vi "Application Example Advanced with Debug.vi"() -> ()   [LabVIEW 2019]
uses:
  <vilib>/addons/Automotive Diagnostic Command Set/NI_Automotive Diagnostic Command Set.lvlib
  Engine/SubVIs/GMLAN/GMLAN.lvlib
  Engine/SubVIs/GMLAN/_SubVIs/ReadDiagnosticInformation_ByStatus.vi
  <vilib>/xnet/xnet.llb/XNET Frame Type CAN.ctl
  <vilib>/xnet/xnet.llb/XNET Frame CAN.ctl
  <vilib>/Automotive Diagnostic Command Set/Diagnostic Transport.llb/Property ID.ctl
  Engine/SubVIs/GMLAN/_SubVIs/ReadDataByPacketIdentifier_SubFunctions.ctl
  <vilib>/Automotive Diagnostic Command Set/Diagnostic Transport.llb/Transport Protocol Selector.ctl
  Engine/SubVIs/GMLAN/_SubVIs/DisableNormalCommunication_Parameter.ctl
  <vilib>/xnet/xnet.llb/XNET Database Close (Database).vi
  <vilib>/xnet/xnet.llb/XNET Read (Frame CAN).vi
  <vilib>/xnet/xnet.llb/XNET Create Session (Frame Input Queued).vi
  <vilib>/Automotive Diagnostic Command Set/Diagnostic Protocols.llb/Diagnostic Trouble Code.ctl
  <vilib>/Automotive Diagnostic Command Set/Diagnostic Transport.llb/Diag CAN Frame Log.ctl
  <resource>/objmgr/xnet.rc
  _SubVIs/CAN Frame.ctl
  <vilib>/Automotive Diagnostic Command Set/Diagnostic Protocols.llb/DTC Descriptor.ctl
  _SubVIs/DPID Periodic Rate.ctl
  _SubVIs/DPID Parameters.ctl
  Engine/SubVIs/GMLAN/_SubVIs/DTCStatusMask.ctl
panel:
  in  "Enable Comm":bool
  out "Bus Traffic":string[][](table)=[["09/16/2012 22:50:39.244581", "01\t68\tAA\tAA\tAA\tAA\tAA\tAA\r\n", "000007E8", "CAN Data", "No", "No"], ["09/16/2012 22:50:39.235716", "ED\t40\t00\t0F\t38\t00\t83\tFD\r\n", "000001F5", "CAN Data", "No", "No"], ["09/16/2012 22:50:39.235476", "6D\t02\tC0\t30\r\n", "000001C4", "CAN Data", "No", "No"], ["09/16/2012 22:50:39.235306", "06\t45\t07\t06\t00\t00\t00\t00\r\n", "000001C3", "CAN Data", "No", "No"], ["09/16/2012 22:50:39.234921", "00\t00\t00\t00\r\n", "000001EF", "CAN Data", "No", "No"], ["09/16/2012 22:50:39.234745", "01\t90\t00\t00\t00\t00\t00\t00\r\n", "000001ED", "CAN Data", "No", "No"], ["09/16/2012 22:50:39.234497", "00\t00\t00\t0D\t00\t10\t00\t00\r\n", "000000C9", "CAN Data", "No", "No"], ["09/16/2012 22:50:39.222361", "00\t00\t00\t00\r\n", "000001EF", "CAN Data", "No", "No"], ["09/16/2012 22:50:39.222179", "01\t90\t00\t00\t00\t00\t00\t00\r\n", "000001ED", "CAN Data", "No", "No"], ["09/16/2012 22:50:39.221930", "00\t00\t00\t0A\t00\t10\t00\t00\r\n", "000000C9", "CAN Data", "No", "No"], ["09/16/2012 22:50:39.211623", "00\t00\t00\t00\t00\t00\t00\t00\r\n", "000003E9", "CAN Data", "No", "No"], ["09/16/2012 22:50:39.211370", "01\t34\t00\t00\t00\t00\t00\t00\r\n", "000003D1", "CAN Data", "No", "No"], ["09/16/2012 22:50:39.211122", "07\t65\t08\t04\t00\t00\t00\t00\r\n", "000003C1", "CAN Data", "No", "No"], ["09/16/2012 22:50:39.210879", "06\t45\t06\tA0\t06\tA0\tA9\r\n", "000002C3", "CAN Data", "No", "No"], ["09/16/2012 22:50:39.210661", "ED\t40\t00\t0F\t38\t00\t83\tFD\r\n", "000001F5", "CAN Data", "No", "No"], ["09/16/2012 22:50:39.210421", "4A\t02\tC0\t30\r\n", "000001C4", "CAN Data", "No", "No"], ["09/16/2012 22:50:39.210252", "06\t45\t07\t06\t00\t00\t00\t00\r\n", "000001C3", "CAN Data", "No", "No"], ["09/16/2012 22:50:39.209862", "00\t00\t00\t00\r\n", "000001EF", "CAN Data", "No", "No"], ["09/16/2012 22:50:39.209686", "01\t90\t00\t00\t00\t00\t00\t00\r\n", "000001ED", "CAN Data", "No", "No"], ["09/16/2012 22:50:39.209438", "00\t00\t00\t07\t00\t10\t00\t00\r\n", "000000C9", "CAN Data", "No", "No"], ["09/16/2012 22:50:39.197360", "00\t00\t00\t00\r\n", "000001EF", "CAN Data", "No", "No"], ["09/16/2012 22:50:39.197180", "01\t90\t00\t00\t00\t00\t00\t00\r\n", "000001ED", "CAN Data", "No", "No"], ["09/16/2012 22:50:39.196931", "00\t00\t00\t00\t00\t10\t00\t00\r\n", "000000C9", "CAN Data", "No", "No"], ["09/16/2012 22:50:39.185679", "ED\t40\t00\t0F\t38\t00\t83\tFD\r\n", "000001F5", "CAN Data", "No", "No"], ["09/16/2012 22:50:39.185439", "27\t02\tC0\t30\r\n", "000001C4", "CAN Data", "No", "No"], ["09/16/2012 22:50:39.185273", "06\t45\t07\t06\t00\t00\t00\t00\r\n", "000001C3", "CAN Data", "No", "No"], ["09/16/2012 22:50:39.184882", "00\t00\t00\t00\r\n", "000001EF", "CAN Data", "No", "No"], ["09/16/2012 22:50:39.184708", "01\t90\t00\t00\t00\t00\t00\t00\r\n", "000001ED", "CAN Data", "No", "No"], ["09/16/2012 22:50:39.184460", "00\t00\t00\t0D\t00\t10\t00\t00\r\n", "000000C9", "CAN Data", "No", "No"], ["09/16/2012 22:50:39.172360", "00\t00\t00\t00\r\n", "000001EF", "CAN Data", "No", "No"], ["09/16/2012 22:50:39.172178", "01\t90\t00\t00\t00\t00\t00\t00\r\n", "000001ED", "CAN Data", "No", "No"], ["09/16/2012 22:50:39.171929", "00\t00\t00\t0A\t00\t10\t00\t00\r\n", "000000C9", "CAN Data", "No", "No"], ["09/16/2012 22:50:39.160898", "06\t45\t06\tA0\t06\tA0\tA9\r\n", "000002C3", "CAN Data", "No", "No"], ["09/16/2012 22:50:39.160679", "ED\t40\t00\t0F\t38\t00\t83\tFD\r\n", "000001F5", "CAN Data", "No", "No"], ["09/16/2012 22:50:39.160439", "00\t02\tC0\t30\r\n", "000001C4", "CAN Data", "No", "No"], ["09/16/2012 22:50:39.160263", "06\t45\t07\t06\t00\t00\t00\t00\r\n", "000001C3", "CAN Data", "No", "No"], ["09/16/2012 22:50:39.159870", "00\t00\t00\t00\r\n", "000001EF", "CAN Data", "No", "No"], ["09/16/2012 22:50:39.159696", "01\t90\t00\t00\t00\t00\t00\t00\r\n", "000001ED", "CAN Data", "No", "No"], ["09/16/2012 22:50:39.159448", "00\t00\t00\t07\t00\t10\t00\t00\r\n", "000000C9", "CAN Data", "No", "No"], ["09/16/2012 22:50:39.147362", "00\t00\t00\t00\r\n", "000001EF", "CAN Data", "No", "No"], ["09/16/2012 22:50:39.147180", "01\t90\t00\t00\t00\t00\t00\t00\r\n", "000001ED", "CAN Data", "No", "No"], ["09/16/2012 22:50:39.146932", "00\t00\t00\t00\t00\t10\t00\t00\r\n", "000000C9", "CAN Data", "No", "No"], ["09/16/2012 22:50:39.135714", "ED\t40\t00\t0F\t38\t00\t83\tFD\r\n", "000001F5", "CAN Data", "No", "No"], ["09/16/2012 22:50:39.135473", "6D\t02\tC0\t30\r\n", "000001C4", "CAN Data", "No", "No"], ["09/16/2012 22:50:39.135303", "06\t45\t07\t06\t00\t00\t00\t00\r\n", "000001C3", "CAN Data", "No", "No"], ["09/16/2012 22:50:39.134917", "00\t00\t00\t00\r\n", "000001EF", "CAN Data", "No", "No"], ["09/16/2012 22:50:39.134741", "01\t90\t00\t00\t00\t00\t00\t00\r\n", "000001ED", "CAN Data", "No", "No"], ["09/16/2012 22:50:39.134492", "00\t00\t00\t0D\t00\t10\t00\t00\r\n", "000000C9", "CAN Data", "No", "No"], ["09/16/2012 22:50:39.122361", "00\t00\t00\t00\r\n", "000001EF", "CAN Data", "No", "No"], ["09/16/2012 22:50:39.122180", "01\t90\t00\t00\t00\t00\t00\t00\r\n", "000001ED", "CAN Data", "No", "No"]]
  out "Diagnostics Traffic":string[][](table)
  in  "Flush Queue":bool
  in  "Clear Screen":bool
  out "Success?":bool=TRUE
  in  "Read DID":bool
  in  "Read PIDs":bool
  in  "Stop DPIDs":bool
  in  "Start DPIDs":bool
  in  "DTC Reset":bool
  in  "Read DTCs":bool
  in  "Setup DPIDs":bool
  in  "Enable Comm":bool
  in  "Write CPID":bool
  in  "Disable Comm":bool
  in  "Tab Control":T1(tab)
  in  "HW select":u16(ring) items=["NI-XNET", "NI-CAN"]
  in  "CAN Interface":string(combo)="CAN1"
  in  "Baudrate":u32=500000
  in  "Receive ID":u32=2024 format="%.0x"
  in  "Transmit ID":u32=2016 format="%.0x"
  in  "UUDT Receive ID":u32=1512 format="%.0x"
  in  "DPIDs":T3(array[cluster])=[{"DPID ID"=239, "Speed"=enum."Medium", "PIDs"=[14]}, {"DPID ID"=253, "Speed"=enum."Fast", "PIDs"=[12]}] {"PIDs" format="%.0x"; "DPID ID" format="%.0x"}
  in  "DTC descriptor":T4={"DTC Byte Length"=2, "Status Byte Length"=1, "Add Data Byte Length"=1, "Byte Order"=enum."Motorola"}
  in  "DID ID":u8=153 format="%.0x"
  out "DID Data":u8[](array[numeric])=[32, 8, 18, 17]
  out "PID Data":u8[](array[numeric])=[128]
  in  "PID ID":u16=14 format="%.0x"
  in  "CPID ID":u8=29 format="%.0x"
  in  "CPIDControlBytes":u8[](array[numeric])=[0, 0, 0, 0, 0] format="%.0x"
  out "DPID":T5={"DPID ID"=253, "Speed"=enum."Fast", "PIDs"=[12]}
  out "timestamp":timestamp=timestamp(3432175878.295675 s since 1904-01-01)
  out "payload":u8[](array[numeric])
  out "EndofDTCReport":bool=TRUE
  out "DTCs":T6[](array[typedef])
  in  "status mask":T7={"DTC supported by calibration"=FALSE, "current DTC"=TRUE, "test not passed since DTC cleared"=FALSE, "test failed since DTC cleared"=FALSE, "history DTC"=FALSE, "test not passed since current power up"=FALSE, "current DTC since power up"=FALSE, "warning indicator requested state"=FALSE}
  out "error IO":errorcluster
  in  "stop":bool
  out "stopped?":bool=TRUE
  # "$90 - VehicleIdentificationNumber (VIN)\n$92\t- System Supplier ID\n$97\t- SystemNameOrEngineType"
  # "$C - Engine Speed\n$E\t- Spark Advance"
  # "x10 CDAR\nx1D PHSR"
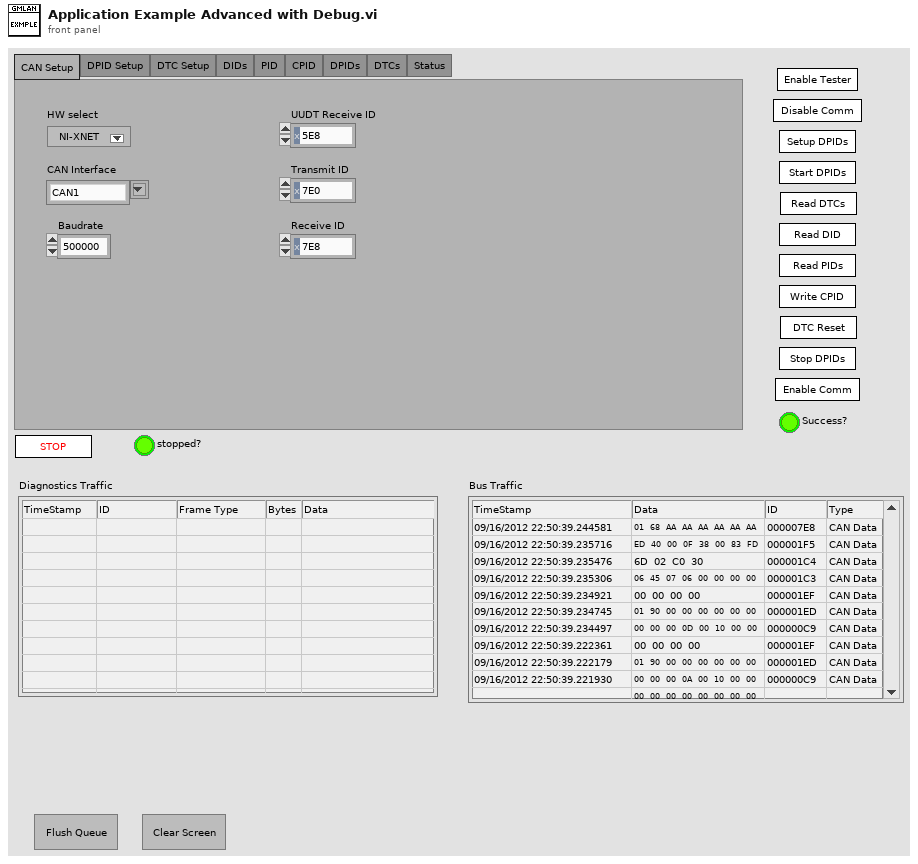
[diagram p1: front panel]
types:
  T1 = enum32{"CAN Setup", "DPID Setup", "DTC Setup", "DIDs", "PID", "CPID", "DPIDs", "DTCs", "Status"}
  T2 = typedef "DPID Periodic Rate.ctl" = enum16{"Slow", "Medium", "Fast"}
  T3 = cluster{"DPID ID":u8, "Speed":T2, "PIDs":u16[]}[]
  T4 = typedef "DTC Descriptor.ctl" = cluster{"DTC Byte Length":i32, "Status Byte Length":i32, "Add Data Byte Length":i32, "Byte Order":enum16{"Motorola", "Intel"}}
  T5 = typedef "DPID Parameters.ctl" = cluster{"DPID ID":u8, "Speed":T2, "PIDs":u16[]}
  T6 = typedef "Diagnostic Trouble Code.ctl" = cluster{"DTC":u32, "Status":u32, "Add Data":u32}
  T7 = typedef "GMLAN.lvlib/DTCStatusMask.ctl" = cluster{"DTC supported by calibration":bool, "current DTC":bool, "test not passed since DTC cleared":bool, "test failed since DTC cleared":bool, "history DTC":bool, "test not passed since current power up":bool, "current DTC since power up":bool, "warning indicator requested state":bool}
  T8 = typedef "CAN Frame.ctl" = cluster{"Frame name":string, "Identifier":u32, "Payload Length":u32, "Timing Type":u32, "Transmit Time":dbl, "Extended Identifier?":bool, "Comment":string}
  T9 = typedef "NI_Automotive Diagnostic Command Set.lvlib/Diag CAN Frame Log.ctl" = cluster{"Timestamp":dbl, "ArbitrationId":u32, "IsRemote":u8, "DataLength":u8, "Data":u8[]}
  T10 = typedef "XNET Frame CAN.ctl" = cluster{"timestamp":timestamp, "payload":u8[], "identifier":u32, "type":T11, "extended?":bool, "echo?":bool}
  T11 = typedef "XNET Frame Type CAN.ctl" = u8
  T12 = typedef "NI_Automotive Diagnostic Command Set.lvlib/Property ID.ctl" = enum16{"Timeout Diag Command", "Timeout FC (Bs)", "Timeout CF (Cr)", "Receive Block Size (BS)", "Wait Time CF (STmin)", "Max Wait Frames (N_WFTmax)", "Wait Frames to Send (N_WAIT)", "Time between Waits (T_W)", "Fill CAN Frames", "Fill Byte", "Invalid Response as Error", "Max RspPending Count", "VWTP Command Timeout", "STmin", "P2min", "Termination", "Timeout RspPending", "LIN Sleep", "Actual CAN IO Mode", "Response Plausibility Check", "Session-based Properties"}
  T13 = typedef "NI_Automotive Diagnostic Command Set.lvlib/Transport Protocol Selector.ctl" = enum16{"ISO TP - Normal Mode", "ISO TP - Mixed Mode", "VW TP 2.0", "Diagnostics on IP", "ISO TP LIN"}
  T14 = typedef "NI_Automotive Diagnostic Command Set.lvlib/Diag Reference.ctl" = cluster{"Diag CAN Handle":u32, "Transport Protocol":T13, "Receive Address Extension":u8, "Transmit Address Extension":u8, "Receive CAN Id":u32, "Transmit CAN Id":u32, "Log Frames ?":bool, "My TP Address":u8, "Other TP Address":u8, "T1":u16, "T2":u16, "T3":u16, "T4":u16, "Tx SN":u8, "Block Size":u8, "Rx SN":u8, "VW TP Initialized?":bool, "Tx block no":u8, "baud rate":u64, "Interface":string, "Channel Diag CAN Handle":u32, "UDP Connection ID":refnum<k16>, "TCP Connection ID":refnum<k5>, "Target IP Addr":u32, "Source Address":u16, "Target Address":u16, "Send Header NACK?":bool, "DLL Handle":u32, "NAD":u8, "Time Stamp read first":dbl, "Time Stamp read last":dbl, "Time Stamp write first":dbl, "Time Stamp write last":dbl, "Time Stamp write":dbl, "Time Stamp read":dbl, " I/O Mode":u32, "FD Baudrate":u64, "TX_DL":u16, "RX_DL":u16, "DoIP Protocol Version":T15, " Selected I/O Mode":u32, "TesterPresent Counter":u32, "TesterPresent Limit":u32, "TesterPresent Tick[ms]":i32, "TesterPresent RequireResponse?":bool, "TesterPresent Stored Ref?":bool, "TesterPresent Message":u8[], "TesterPresent Task Handle":i32, "TesterPresent Semaphore":T16, "Response Plausibility Check":u32, "Default Version?":bool, "Diagostic Globals":T17, "Session-based Properties?":bool}
  T15 = typedef "NI_Automotive Diagnostic Command Set.lvlib/DoIP Protocol Version.ctl" = u8
  T16 = typedef "Semaphore RefNum" = refnum<k1>
  T17 = typedef "NI_Automotive Diagnostic Command Set.lvlib/Diag Globals.ctl" = cluster{"Timeout FC (Bs)":u32, "Timeout CF (Cr)":u32, "Timeout Diag Command":u32, "Receive Block Size (BS)":u8, "Wait Time CF (STmin)":u8, "Max Waits (N_WFTmax)":u8, "Waits to Send (N_WAIT)":i32, "Time between Waits (TW)":u32, "Fill CAN Frames?":bool, "Fill Byte":u32, "Invalid Response as Error?":bool, "Max RspPending Count":u32, "VWTP Command Timeout":u32, "Transport Protocol":T13, "Diag CAN Handle":u32, "DLL Handle":u32, "Timeout RspPending":u32}
  T18 = enum8{"Idle", "Read DID", "Read DTCs", "Reset DTCs", "Setup DPIDs", "Start DPIDs", "Stop DPIDs", "Read PID", "Write CPID", "DisableCommunication", "EnableCommunication", "Stop"}
  T19 = typedef "GMLAN.lvlib/ReadDataByPacketIdentifier_SubFunctions.ctl" = enum8{"stopSending", "sendOneResponse", "scheduleAtSlowRate", "scheduleAtMediumRate", "scheduleAtFastRate"}
  T20 = typedef "GMLAN.lvlib/DisableNormalCommunication_Parameter.ctl" = enum8{"SpecificECU", "EntireNetwork"}
  T21 = typedef "Filtered DPID IDs.ctl" = cluster{"Slow":u8[], "Medium":u8[], "Fast":u8[]}
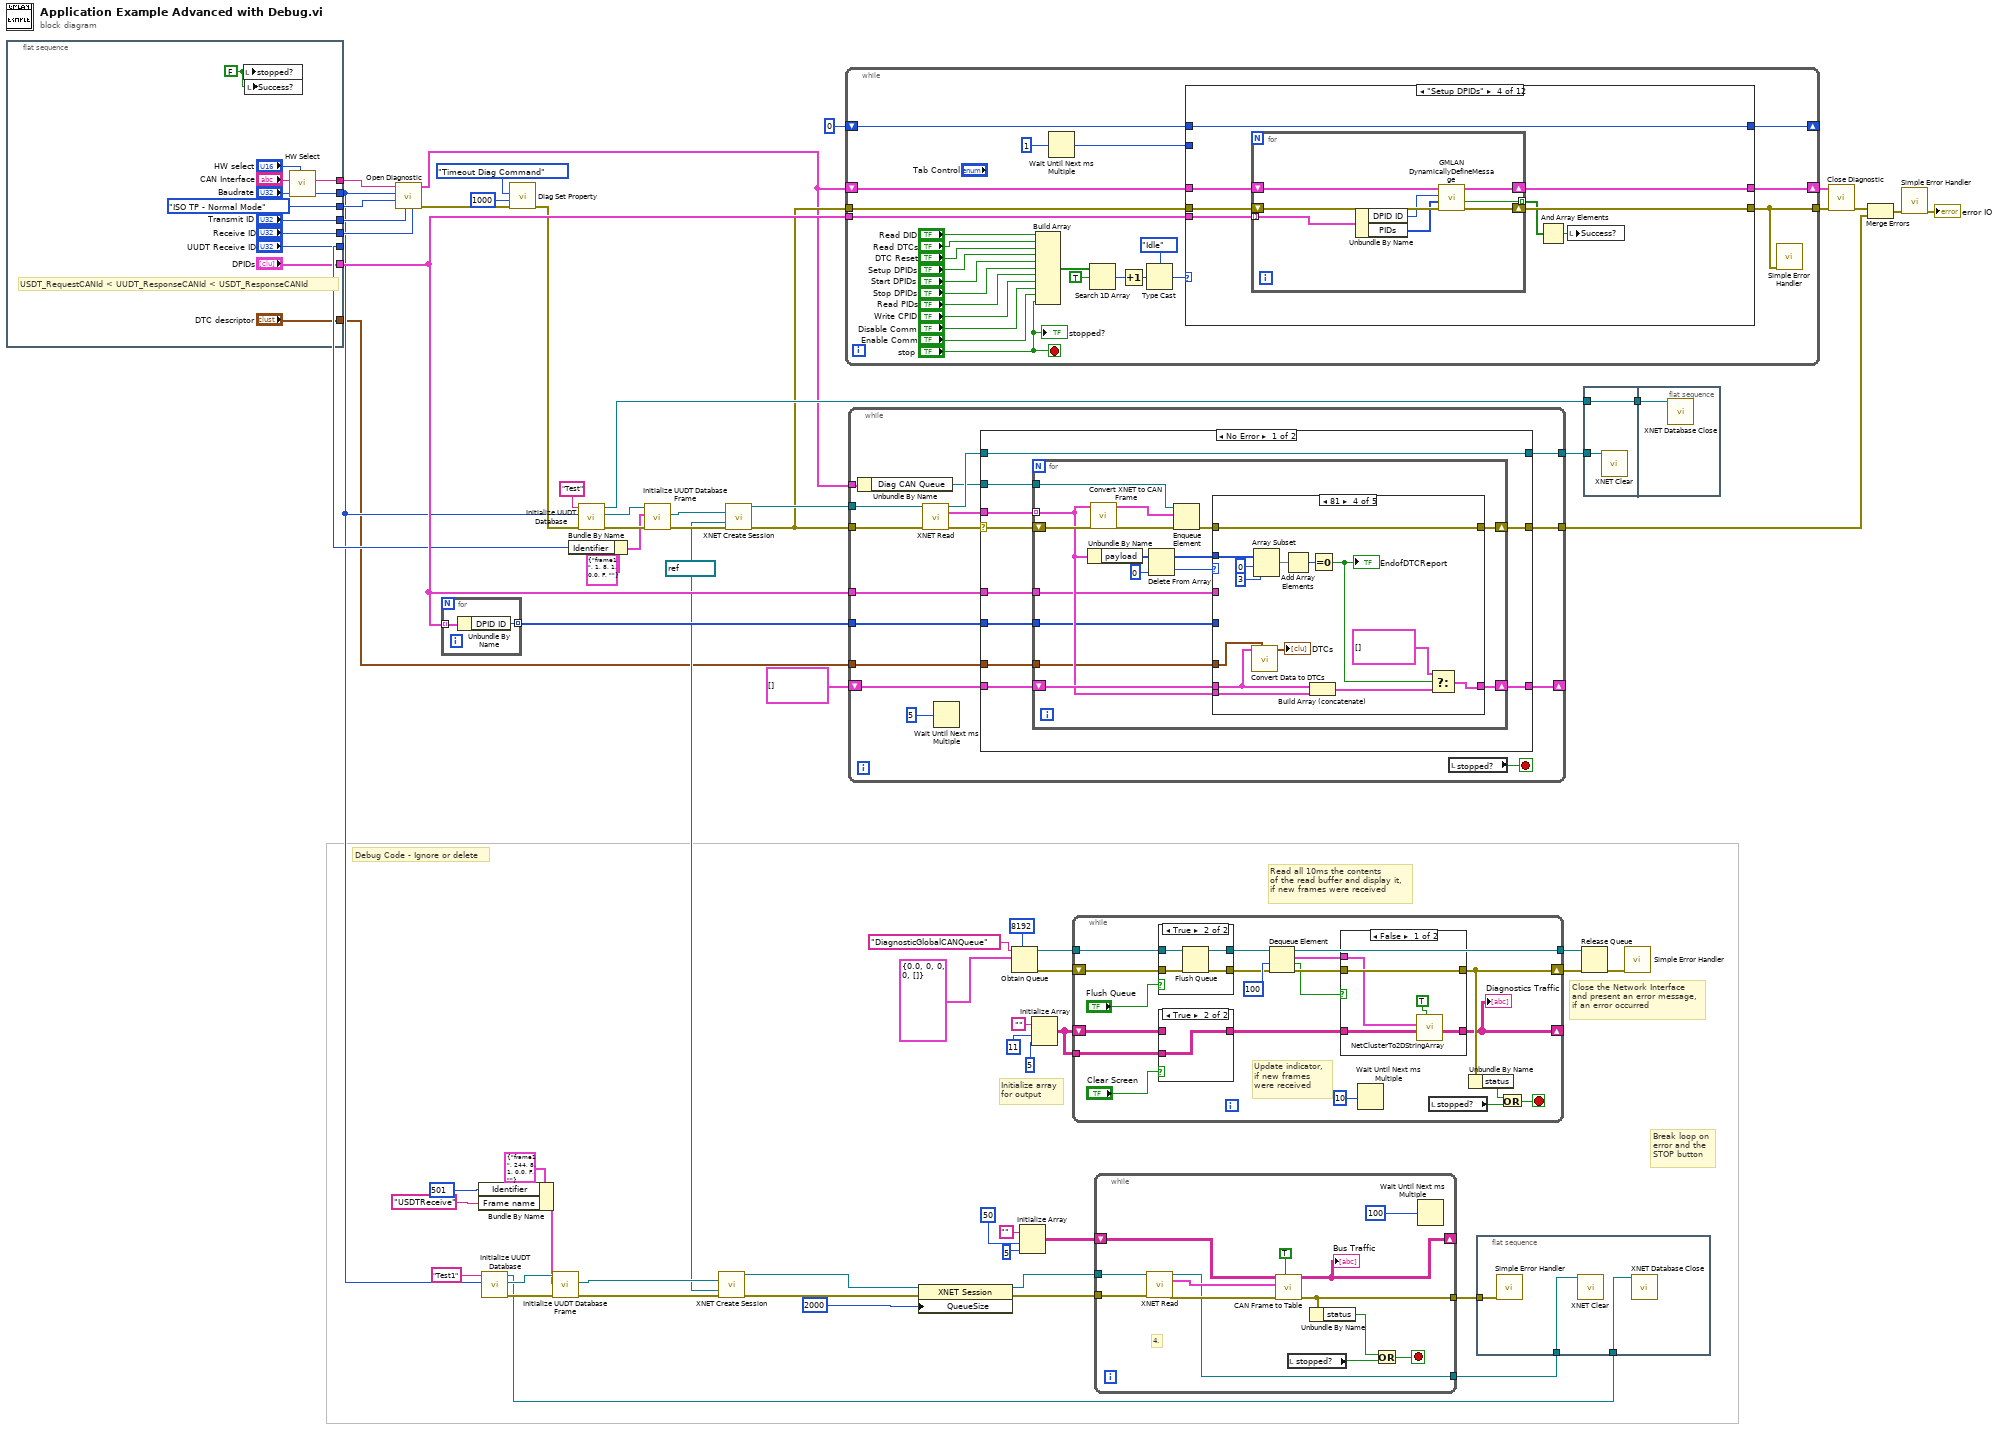
[diagram p0: block diagram]
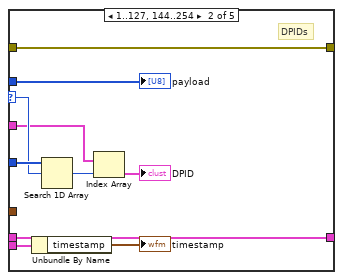
[diagram p6: hidden frame]
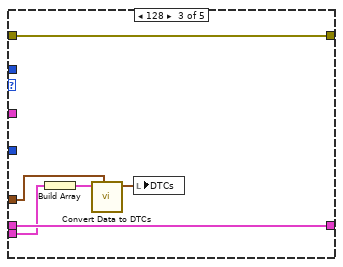
[diagram p7: hidden frame]
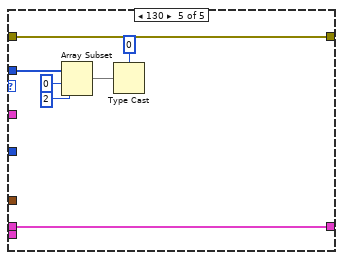
[diagram p8: hidden frame]
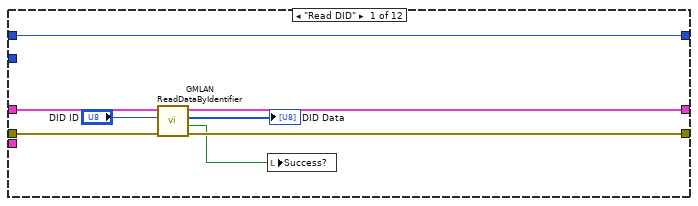
[diagram p10: hidden frame]
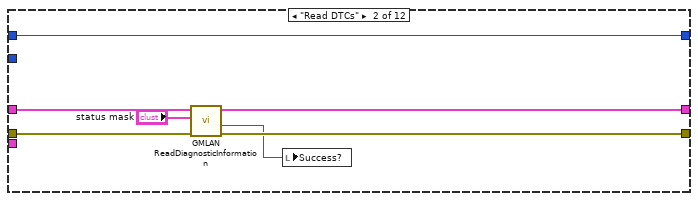
[diagram p11: hidden frame]
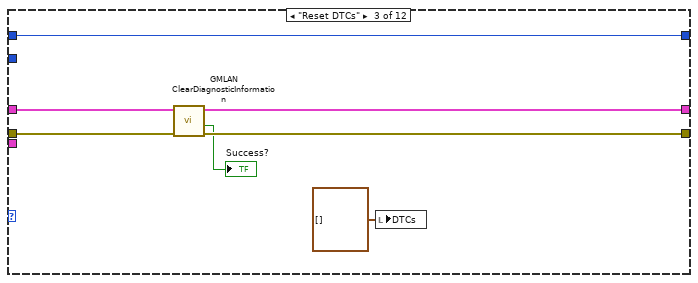
[diagram p12: hidden frame]
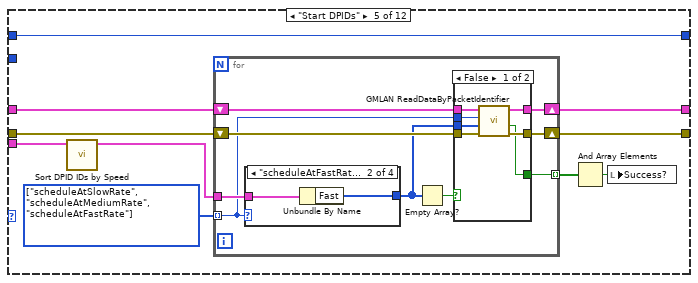
[diagram p13: hidden frame]
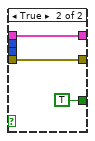
[diagram p14: hidden frame]
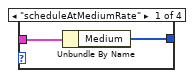
[diagram p15: hidden frame]
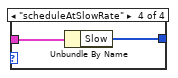
[diagram p17: hidden frame]
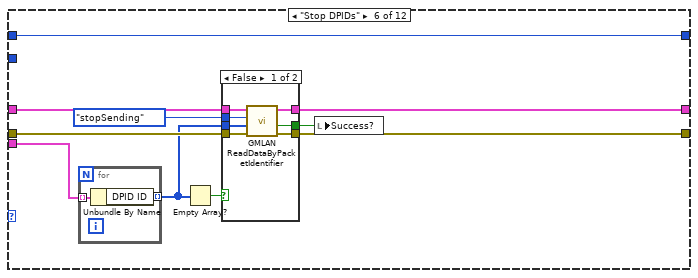
[diagram p18: hidden frame]
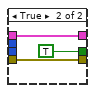
[diagram p19: hidden frame]
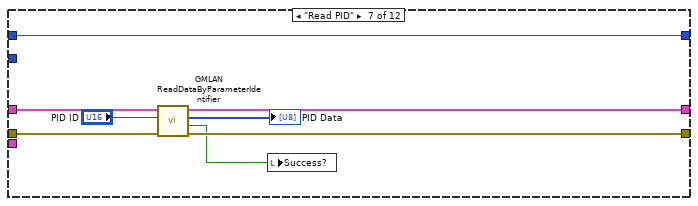
[diagram p20: hidden frame]
diagram:
  w3 = refnum<k21> "CAN1" ("interface")
  # "Debug Code - Ignore or delete"
  # "Break loop on \nerror and the \nSTOP button"
  # "Initialize array \nfor output"
  # "Close the Network Interface \nand present an error message, \nif an error occurred"
  # "Read all 10ms the contents \nof the read buffer and display it, \nif new frames were received"
  n1 = flat-sequence {
    tunnel: [w79] -> w66
    tunnel: ["Baudrate"] -> w2
    tunnel: [Transport_Protocol_Selector."ISO TP - Normal Mode" ("Transport Protocol")] -> w65
    tunnel: ["Transmit ID"] -> w64
    tunnel: ["Receive ID"] -> w63
    tunnel: ["UUDT Receive ID"] -> w44
    tunnel: ["DTC descriptor"] -> w1
    tunnel: ["DPIDs"] -> w53
    frame #0 {
      w69 = FALSE ("stopped?")
      # "USDT_RequestCANId < UUDT_ResponseCANId < USDT_ResponseCANId"
      n2 = local write "stopped?"(w69) -> ()
      n3 = local write "Success?"(w69) -> ()
      n4 = call "HW Select.vi"("HW select"="HW select", "CAN port"="CAN Interface") -> ("CAN port out"=w79:string)  [unwired: 9 in]
    }
  }
  n5 = call <vilib>:"Open Diagnostic.vi"("Receive ID"=w63, "Transmit ID"=w64, "Transport Protocol"=w65, "Baud Rate"=w2, "CAN Interface"=w66) -> ("error out"=w62:errorcluster, "diag ref out"=w37:T14)  [unwired: 1 in, 4 out]
  n6 = for {
    tunnel: w53 -> [w81] mode=indexing
    tunnel: [w80] -> w59 mode=indexing
    n7 = Unbundle By Name(w81) -> ("DPID ID"=w80:u8)
  }
  n8 = Bundle By Name(cluster=T8 {"Frame name"="frame1", "Identifier"=244, "Payload Length"=8, "Timing Type"=1, "Transmit Time"=0.0, "Extended Identifier?"=FALSE, "Comment"=""} ("CAN Frame"), "Identifier"=u32 501 ("UUDT Receive ID"), "Frame name"="USDTReceive") -> (w8:T8)
  n9 = call "Initialize UUDT Database.vi"("Baud Rate"=w2, "Addon Name"="Test1") -> ("error out"=w10:errorcluster, "Cluster"=w9:refnum<k21>, "XNET Database"=w6:refnum<k21>)  [unwired: 7 in]
  n10 = call <vilib>:"Diag Set Property.vi"("error in (no error)"=w62, "property value"=u32 1000, "property ID"=Property_ID."Timeout Diag Command") -> ("error out"=w39:errorcluster)  [unwired: 7 in, 1 out]
  n11 = call "Initialize UUDT Database Frame.vi"("error in"=w10, "CAN Frame"=w8, "cluster in"=w9) -> ("error out"=w7:errorcluster, "frame out"=w4:refnum<k21>)  [unwired: 6 in, 1 out]
  n12 = Bundle By Name(cluster=T8 {"Frame name"="frame1", "Identifier"=1, "Payload Length"=8, "Timing Type"=1, "Transmit Time"=0.0, "Extended Identifier?"=FALSE, "Comment"=""} ("CAN Frame"), "Identifier"=w44) -> (w42:T8)
  n13 = call "Initialize UUDT Database.vi"("error in (no error)"=w39, "Baud Rate"=w2, "Addon Name"="Test") -> ("error out"=w49:errorcluster, "Cluster"=w48:refnum<k21>, "XNET Database"=w40:refnum<k21>)  [unwired: 6 in]
  n14 = call "Initialize UUDT Database Frame.vi"("error in"=w49, "CAN Frame"=w42, "cluster in"=w48) -> ("error out"=w46:errorcluster, "frame out"=w47:refnum<k21>)  [unwired: 6 in, 1 out]
  n15 = call-poly <vilib>:"XNET Create Session.vi"("frame"=w4, "interface"=w3, "error in (no error)"=w7) -> ("session out"=w17:refnum<k21>, "error out"=w13:errorcluster)  [unwired: 11 out]
  n16 = call-poly <vilib>:"XNET Create Session.vi"("frame"=w47, "interface"=w3, "error in (no error)"=w46) -> ("session out"=w50:refnum<k21>, "error out"=w38:errorcluster)  [unwired: 11 out]
  n17 = while {
    tunnel: w38 -> [w106]
    tunnel: [w85] -> w67
    shift-right: [w105] -> w68
    shift-left: w37 -> [w107]
    shift-right: [w99] -> _
    shift-left: u32 0 ("millisecond timer value") -> [w97]
    tunnel: w53 -> [w93]
    stop <- "stop" stop-if-true
    n18 = Build Array("Read DID", "Read DTCs", "DTC Reset", "Setup DPIDs", "Start DPIDs", "Stop DPIDs", "Read PIDs", "Write CPID", "Disable Comm", "Enable Comm", "stop") -> (w103:bool[])
    n19 = Wait Until Next ms Multiple(millisecond multiple=1) -> (millisecond timer value=w98:u32)
    n20 = Search 1D Array(1D array=w103, element=TRUE) -> (index of element=w90:i32)  [unwired: 1 in]
    n21 = Increment(x=w90) -> (x+1=w88:u8)
    n22 = Type Cast(type=T18."Idle", x=w88) -> (*(type *) &x=w87:T18)
    n23 = case shown="\"Setup DPIDs\"" w87 {
      tunnel: w107 -> [w115 w121 w129 w134 w153 w188 w210 w217 w224 w230 w232 w245]
      tunnel: w106 -> [w114 w119 w128 w136 w155 w190 w209 w218 w225 w231 w233 w246]
      tunnel: [w113 w117 w127 w133 w152 w187 w208 w215 w222 w228 w232 w243] -> w105
      tunnel: [w112 w118 w126 w135 w154 w189 w207 w216 w223 w229 w233 w244] -> w85
      tunnel: w98 -> [_ _ _ _ _ _ _ _ _ _ _ w241]
      tunnel: [w108 w122 w125 w137 w151 w186 w203 w214 w221 w227 w234 w242] -> w99
      tunnel: w97 -> [w108 w122 w125 w137 w151 w186 w203 w214 w221 w227 w234 w237]
      tunnel: w93 -> [_ _ _ w132 w150 w185 _ _ _ _ _ _]
      frame "Read DID" {
        n24 = call "GMLAN ReadDataByIdentifier.vi"("error in (no error)"=w114, "Data ID (DID)"="DID ID", "diag ref in"=w115) -> ("error out"=w112:errorcluster, "success?"=w111:bool, "data out"=→"DID Data":u8[], "diag ref out"=w113:T14)  [unwired: 5 in]
        n25 = local write "Success?"(w111) -> ()
      }
      frame "Read DTCs" {
        n26 = call-poly "GMLAN ReadDiagnosticInformation.vi"("error in (no error)"=w119, "status mask"="status mask", "diag ref in"=w121) -> ("error out"=w118:errorcluster, "success?"=w116:bool, "diag ref out"=w117:T14)  [unwired: 5 in, 1 out]
        n27 = local write "Success?"(w116) -> ()
      }
      frame "Reset DTCs" {
        n28 = call "GMLAN ClearDiagnosticInformation.vi"("error in (no error)"=w128, "diag ref in"=w129) -> ("error out"=w126:errorcluster, "success?"=→"Success?":bool, "diag ref out"=w127:T14)  [unwired: 7 in]
        n29 = local write "DTCs"(T6[] [] ("DTCs")) -> ()
      }
      frame "Setup DPIDs" {
        n30 = for {
          shift-right: [w144] -> w135
          shift-left: w136 -> [w145]
          shift-right: [w142] -> w133
          shift-left: w134 -> [w143]
          tunnel: w132 -> [w141] mode=indexing
          tunnel: [w138] -> w131 mode=indexing
          n31 = Unbundle By Name(w141) -> ("DPID ID"=w140:u8, "PIDs"=w139:u16[])
          n32 = call "GMLAN DynamicallyDefineMessage.vi"("error in (no error)"=w145, "PID List"=w139, "DPID ID"=w140, "diag ref in"=w143) -> ("error out"=w144:errorcluster, "success?"=w138:bool, "diag ref out"=w142:T14)  [unwired: 5 in]
        }
        n33 = And Array Elements(Boolean array=w131) -> (logical AND=w130:bool)
        n34 = local write "Success?"(w130) -> ()
      }
      frame "Start DPIDs" {
        w148 = T19[] [enum."scheduleAtSlowRate", enum."scheduleAtMediumRate", enum."scheduleAtFastRate"] items=["stopSending", "sendOneResponse", "scheduleAtSlowRate", "scheduleAtMediumRate", "scheduleAtFastRate"]
        n35 = call "Sort DPID IDs by Speed.vi"("DPIDs"=w150) -> ("Filtered DPIDs IDs"=w149:T21)  [unwired: 10 in]
        n36 = for {
          tunnel: w149 -> [w160]
          shift-right: [w163] -> w154
          shift-left: w155 -> [w164]
          shift-right: [w161] -> w152
          shift-left: w153 -> [w162]
          tunnel: w148 -> [w157] mode=indexing
          tunnel: [w156] -> w146 mode=indexing
          n37 = case shown="\"scheduleAtFastRate\"" w157 {
            tunnel: w160 -> [w176 w178 _ w180]
            tunnel: [w175 w177 _ w179] -> w159
            frame "scheduleAtMediumRate" {
              n38 = Unbundle By Name(w176) -> ("Medium"=w175:u8[])
            }
            frame "scheduleAtFastRate" {
              n39 = Unbundle By Name(w178) -> ("Fast"=w177:u8[])
            }
            frame Default {
            }
            frame "scheduleAtSlowRate" {
              n40 = Unbundle By Name(w180) -> ("Slow"=w179:u8[])
            }
          }
          n41 = Empty Array?(array=w159) -> (empty?=w158:bool)
          n42 = case shown="False" w158 {
            tunnel: w164 -> [w171 w173]
            tunnel: [w170 w173] -> w163
            tunnel: w162 -> [w169 w174]
            tunnel: [w168 w174] -> w161
            tunnel: w157 -> [w167 _]
            tunnel: w159 -> [w166 _]
            tunnel: [w165 TRUE ("success?")] -> w156
            frame False {
              n43 = call "GMLAN ReadDataByPacketIdentifier.vi"("error in (no error)"=w171, "DPIDs"=w166, "Sub Function"=w167, "diag ref in"=w169) -> ("error out"=w170:errorcluster, "success?"=w165:bool, "diag ref out"=w168:T14)  [unwired: 4 in, 1 out]
            }
            frame True {
            }
          }
        }
        n44 = And Array Elements(Boolean array=w146) -> (logical AND=w147:bool)
        n45 = local write "Success?"(w147) -> ()
      }
      frame "Stop DPIDs" {
        n46 = for {
          tunnel: w185 -> [w202] mode=indexing
          tunnel: [w201] -> w183 mode=indexing
          n47 = Unbundle By Name(w202) -> ("DPID ID"=w201:u8)
        }
        n48 = Empty Array?(array=w183) -> (empty?=w184:bool)
        n49 = case shown="False" w184 {
          tunnel: w190 -> [w197 w199]
          tunnel: [w196 w199] -> w189
          tunnel: w188 -> [w195 w200]
          tunnel: [w194 w200] -> w187
          tunnel: ReadDataByPacketIdentifier_SubFunctions."stopSending" ("Sub Function") -> [w193 _]
          tunnel: w183 -> [w192 _]
          tunnel: [w191 TRUE ("success?")] -> w181
          frame False {
            n50 = call "GMLAN ReadDataByPacketIdentifier.vi"("error in (no error)"=w197, "DPIDs"=w192, "Sub Function"=w193, "diag ref in"=w195) -> ("error out"=w196:errorcluster, "success?"=w191:bool, "diag ref out"=w194:T14)  [unwired: 4 in, 1 out]
          }
          frame True {
          }
        }
        n51 = local write "Success?"(w181) -> ()
      }
      frame "Read PID" {
        n52 = call "GMLAN ReadDataByParameterIdentifier.vi"("error in (no error)"=w209, "Parameter ID (PID)"="PID ID", "diag ref in"=w210) -> ("error out"=w207:errorcluster, "success?"=w206:bool, "data out"=→"PID Data":u8[], "diag ref out"=w208:T14)  [unwired: 5 in]
        n53 = local write "Success?"(w206) -> ()
      }
      frame "Write CPID" {
        n54 = call "GMLAN DeviceControl.vi"("error in (no error)"=w218, "CPIDControlBytes"="CPIDControlBytes", "CPID ID"="CPID ID", "diag ref in"=w217) -> ("error out"=w216:errorcluster, "success?"=w213:bool, "diag ref out"=w215:T14)  [unwired: 5 in]
        n55 = local write "Success?"(w213) -> ()
      }
      frame "DisableCommunication" {
        n56 = call "GMLAN DisableNormalCommunication.vi"("error in (no error)"=w225, "Parameter"=DisableNormalCommunication_Parameter."SpecificECU", "diag ref in"=w224) -> ("error out"=w223:errorcluster, "success?"=w219:bool, "diag ref out"=w222:T14)  [unwired: 6 in]
        n57 = local write "Success?"(w219) -> ()
      }
      frame "EnableCommunication" {
        n58 = call "GMLAN ReturnToNormalMode.vi"("error in (no error)"=w231, "diag ref in"=w230) -> ("error out"=w229:errorcluster, "success?"=w226:bool, "diag ref out"=w228:T14)  [unwired: 7 in]
        n59 = local write "Success?"(w226) -> ()
      }
      frame "Stop" {
      }
      frame Default {
        # "Tester Present"
        n60 = Subtract(x=w241, y=w237) -> (x-y=w240:u32)
        n61 = Greater Or Equal?(x=w240, y=u32 1000) -> (x >= y?=w238:bool)
        n62 = Compound Arithmetic op=AND(w238, "Enable Comm") -> (w236:bool)
        n63 = case shown="True" w236 {
          tunnel: w246 -> [w248 w254]
          tunnel: w245 -> [w249 w253]
          tunnel: [w248 w252] -> w244
          tunnel: [w249 w251] -> w243
          tunnel: w241 -> [_ w250]
          tunnel: [w247 w250] -> w242
          tunnel: w237 -> [w247 _]
          frame False {
          }
          frame True {
            n64 = call "GMLAN TesterPresent.vi"("error in (no error)"=w254, "diag ref in"=w253) -> ("error out"=w252:errorcluster, "diag ref out"=w251:T14)  [unwired: 7 in, 1 out]
          }
        }
      }
    }
    n65 = call <vilib>:"Simple Error Handler.vi"("error in (no error)"=w85) -> ()  [unwired: 4 in, 5 out]
    "stopped?" <- "stop"
  }
  n66 = while {
    tunnel: w38 -> [w267]
    shift-right: [w263] -> _
    shift-left: T10[] [] ("data") -> [w264]
    tunnel: w1 -> [w262]
    tunnel: [w260] -> w57
    tunnel: w53 -> [w259]
    tunnel: w59 -> [w258]
    tunnel: w50 -> [w268]
    tunnel: [w257] -> w51
    tunnel: w37 -> [w256]
    stop <- w270 stop-if-true
    n67 = Unbundle By Name(w256) -> ("Diag CAN Queue"=w255:refnum<queue>)
    n68 = call-poly <vilib>:"XNET Read.vi"("session in"=w268, "error in (no error)"=w267) -> ("session out"=w261:refnum<k21>, "data"=w265:T10[], "error out"=w266:errorcluster)  [unwired: 10 in, 1 out]
    n69 = Wait Until Next ms Multiple(millisecond multiple=5) -> ()  [unwired: 1 out]
    n70 = case shown="No Error" w266 {
      selector: w266 -> [w278 w337]
      tunnel: w265 -> [w271 _]
      tunnel: [w277 w337] -> w260
      tunnel: w264 -> [w280 w336]
      tunnel: [w279 w336] -> w263
      tunnel: w255 -> [w276 _]
      tunnel: w262 -> [w275 _]
      tunnel: w261 -> [w272 w335]
      tunnel: w259 -> [w274 _]
      tunnel: w258 -> [w273 _]
      tunnel: [w272 w335] -> w257
      frame No Error {
        n71 = for {
          tunnel: w271 -> [w287] mode=indexing
          shift-right: [w293] -> w279
          shift-left: w280 -> [w294]
          shift-right: [w292] -> w277
          shift-left: w278 -> [w291]
          tunnel: w276 -> [w289]
          tunnel: w275 -> [w285]
          tunnel: w274 -> [w284]
          tunnel: w273 -> [w283]
          n72 = Unbundle By Name(w287) -> ("payload"=w286:u8[])
          n73 = call "Convert XNET to CAN Frame.vi"("XNET frame"=w287) -> ("CAN Frame"=w288:T9)  [unwired: 10 in]
          n74 = Delete From Array(array=w286, index=0) -> (deleted portion=w295:u8, array with subset deleted=w281:u8[])  [unwired: 1 in]
          n75 = Enqueue Element(queue=w289, element=w288, error in (no error)=w291) -> (error out=w290:errorcluster)  [unwired: 1 in, 2 out]
          n76 = case shown="81" w295 {
            selector: w295 -> [_ w305 _ _ _]
            tunnel: w281 -> [_ w298 _ w327 w330]
            tunnel: w294 -> [w297 w307 w313 w314 w334]
            tunnel: w287 -> [_ w301 w311 w321 _]
            tunnel: [w297 w307 w313 w319 w334] -> w293
            tunnel: [w296 w299 w312 w318 w333] -> w292
            tunnel: w290 -> [w296 w299 w312 w318 w333]
            tunnel: w285 -> [_ _ w309 w316 _]
            tunnel: w284 -> [_ w303 _ _ _]
            tunnel: w283 -> [_ w306 _ _ _]
            frame Default {
            }
            frame 1..127, 144..254 {
              # "DPIDs"
              n77 = Unbundle By Name(w301) -> ("timestamp"=→"timestamp":timestamp)
              n78 = Search 1D Array(1D array=w306, element=w305) -> (index of element=w304:i32)  [unwired: 1 in]
              n79 = Index Array(array=w303, index=w304) -> (element=→"DPID":cluster{"DPID ID":u8, "Speed":T2, "PIDs":u16[]})
              "payload" <- w298
            }
            frame 128 {
              n80 = Build Array(w311) -> (w310:T10[])
              n81 = call "Convert Data to DTCs.vi"("DTC descriptor"=w309, "All DTCs"=w310) -> ("DTCs"=w308:T6[])  [unwired: 8 in, 1 out]
              n82 = local write "DTCs"(w308) -> ()
            }
            frame 129 {
              n83 = call "Convert Data to DTCs.vi"("DTC descriptor"=w316, "All DTCs"=w314) -> ("DTCs"=→"DTCs":T6[])  [unwired: 8 in, 1 out]
              n84 = Array Subset(array=w327, index=0, length=3) -> (w324:u8[])
              n85 = Add Array Elements(numeric array=w324) -> (sum=w323:u8)
              n86 = Build Array (concatenate)(w314, w321) -> (w317:T10[])
              n87 = Equal To 0?(x=w323) -> (x = 0?=w322:bool)
              "EndofDTCReport" <- w322
              n88 = Select(t=T10[] [] ("data"), s=w322, f=w317) -> (s? t:f=w319:T10[])
            }
            frame 130 {
              n89 = Array Subset(array=w330, index=0, length=2) -> (w329:u8[])
              n90 = Type Cast(type=u16 0 ("length"), x=w329) -> ()  [unwired: 1 out]
            }
          }
        }
      }
      frame Error {
      }
    }
    n91 = local read "stopped?"() -> (w270:bool)
  }
  n92 = property class="XNET Session"(reference=w17, error in=w13, "QueueSize"=u32 2000 ("Queue Size")) -> (reference out=w16:refnum<k21>, error out=w14:errorcluster)
  n93 = Obtain Queue(max queue size (-1, unlimited)=8192, name (unnamed)="DiagnosticGlobalCANQueue", element data type=T9 {"Timestamp"=0.0, "ArbitrationId"=0, "IsRemote"=0, "DataLength"=0, "Data"=[]} ("CAN FRAME TIMED")) -> (queue out=w31:refnum<queue>, error out=w32:errorcluster)  [unwired: 2 in, 1 out]
  n94 = Initialize Array("", 50 ("Number of Frames to Display"), 5 ("Dimension Size")) -> (w21:string[][])
  n95 = Initialize Array("", 11 ("Dimension Size"), 5 ("Dimension Size")) -> (w25:string[][])
  n96 = while {
    shift-left: w25 -> [w342]
    shift-right: [w353] -> _
    shift-left: w32 -> [w345]
    shift-right: [w355] -> w29
    tunnel: w31 -> [w349]
    tunnel: [w347] -> w30
    tunnel: w25 -> [w339]
    stop <- w354 stop-if-true
    # "Update indicator, \nif new frames \nwere received"
    n97 = case shown="True" "Flush Queue" {
      tunnel: w349 -> [w361 w365]
      tunnel: [w361 w364] -> w346
      tunnel: w345 -> [w360 w363]
      tunnel: [w360 w362] -> w344
      frame False {
      }
      frame True {
        n98 = Flush Queue(queue=w365, error in (no error)=w363) -> (queue out=w364:refnum<queue>, error out=w362:errorcluster)  [unwired: 1 out]
      }
    }
    n99 = case shown="True" "Clear Screen" {
      tunnel: w342 -> [w358 _]
      tunnel: [w358 w359] -> w341
      tunnel: w339 -> [_ w359]
      frame False {
      }
      frame True {
      }
    }
    n100 = Dequeue Element(queue=w346, timeout in ms (-1)=100, error in (no error)=w344) -> (queue out=w347:refnum<queue>, element=w350:T9, timed out?=w351:bool, error out=w352:errorcluster)
    n101 = case shown="False" w351 {
      tunnel: [w368 w371] -> w355
      tunnel: w341 -> [w367 w372]
      tunnel: [w369 w372] -> w353
      tunnel: w352 -> [w368 w371]
      tunnel: w350 -> [w366 _]
      frame False {
        n102 = call <vilib>:"NetClusterTo2DStringArray.vi"("Hexadecimal?"=TRUE, "Input Array"=w367, "Diag Frame"=w366) -> ("Output Array"=w369:string[][])  [unwired: 8 out]
      }
      frame True {
      }
    }
    "Diagnostics Traffic" <- w353
    n103 = Wait Until Next ms Multiple(millisecond multiple=u32 10) -> ()  [unwired: 1 out]
    n104 = local read "stopped?"() -> (w338:bool)
    n105 = Unbundle By Name(w355) -> ("status"=w356:bool)
    n106 = Or(x=w356, y=w338) -> (x .or. y?=w354:bool)
  }
  n107 = while {
    tunnel: w16 -> [w385]
    shift-right: [w375] -> _
    shift-left: w21 -> [w381]
    tunnel: w14 -> [w379]
    tunnel: [w376] -> w12
    tunnel: [w374] -> w5
    stop <- w384 stop-if-true
    # "4."
    n108 = call-poly <vilib>:"XNET Read.vi"("session in"=w385, "error in (no error)"=w379) -> ("session out"=w374:refnum<k21>, "data"=w382:T10[], "error out"=w377:errorcluster)  [unwired: 11 out]
    n109 = call "CAN Frame to Table.vi"("Hexadecimal?"=TRUE, "error in (no error)"=w377, "CAN Frames (from XNET Read)"=w382, "Input Array"=w381) -> ("error out"=w376:errorcluster, "Output Array"=w375:string[][])  [unwired: 6 in]
    "Bus Traffic" <- w375
    n110 = local read "stopped?"() -> (w373:bool)
    n111 = Unbundle By Name(w376) -> ("status"=w378:bool)
    n112 = Or(x=w378, y=w373) -> (x .or. y?=w384:bool)
    n113 = Wait Until Next ms Multiple(millisecond multiple=u32 100) -> ()  [unwired: 1 out]
  }
  n114 = flat-sequence {
    tunnel: w12 -> [w388]
    tunnel: w6 -> [w387]
    tunnel: w5 -> [w386]
    frame #0 {
      n115 = call <vilib>:"Simple Error Handler.vi"("error in (no error)"=w388) -> ()  [unwired: 1 in, 8 out]
      n116 = call <vilib>:"XNET Clear.vi"("session in"=w386) -> ()  [unwired: 14 in, 1 out]
      n117 = call-poly <vilib>:"XNET Database Close.vi"("database in"=w387) -> ()  [unwired: 14 in, 1 out]
    }
  }
  n118 = Release Queue(queue=w30, error in (no error)=w29) -> (error out=w28:errorcluster)  [unwired: 3 out]
  n119 = flat-sequence {
    tunnel: w51 -> [w390]
    tunnel: [w389] -> w41
    tunnel: w40 -> [w389]
    tunnel: w41 -> [w391]
    frame #0 {
      n120 = call <vilib>:"XNET Clear.vi"("session in"=w390) -> ()  [unwired: 14 in, 1 out]
    }
    frame #1 {
      n121 = call-poly <vilib>:"XNET Database Close.vi"("database in"=w391) -> ()  [unwired: 14 in, 1 out]
    }
  }
  n122 = call <vilib>:"Simple Error Handler.vi"("error in (no error)"=w28) -> ()  [unwired: 1 in, 8 out]
  n123 = call <vilib>:"Close Diagnostic.vi"("error in (no error)"=w67, "diag ref in"=w68) -> ("error out"=w58:errorcluster)  [unwired: 9 out]
  n124 = Merge Errors(w58, w57) -> (w56:errorcluster)
  n125 = call <vilib>:"Simple Error Handler.vi"("error in (no error)"=w56) -> ("error out"=→"error IO":errorcluster)  [unwired: 1 in, 7 out]
